vi "Read Roles.vi"(8 "error in (no error)":errorcluster, 11 "NormalGamePlayVSS in":refnum<class "NormalGamePlayVSS.lvclass">) -> (0 "error out":errorcluster, 2 "Roles":T1, 3 "NormalGamePlayVSS out":refnum<class "NormalGamePlayVSS.lvclass">)   [LabVIEW 2020, in "NormalGamePlayVSS.lvclass"]
uses:
  NormalGamePlayVSS.lvclass
  NormalAttackerRoleVSS_class/NormalAttackerRoleVSS.lvclass
  KeeperRoleVSS_class/KeeperRoleVSS.lvclass
  DefenderAreaRoleVSS_class/DefenderAreaRoleVSS.lvclass
  NormalGamePlayVSS.lvclass/NormalGamePlayVSS.ctl
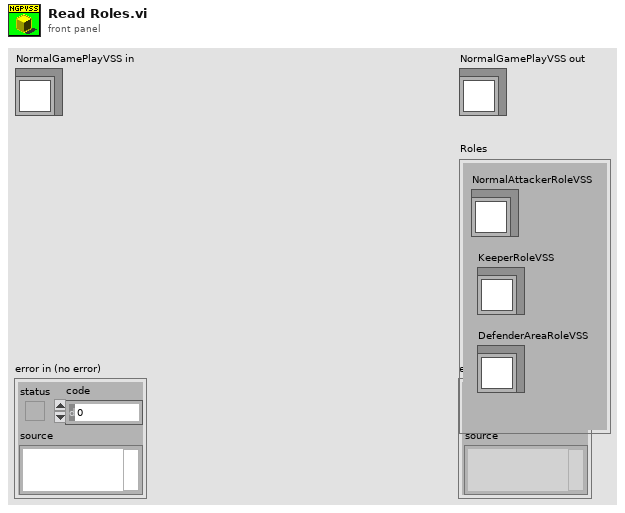
[diagram p1: front panel]
types:
  T1 = cluster{"NormalAttackerRoleVSS":refnum<class "NormalAttackerRoleVSS.lvclass">, "KeeperRoleVSS":refnum<class "KeeperRoleVSS.lvclass">, "DefenderAreaRoleVSS":refnum<class "DefenderAreaRoleVSS.lvclass">}
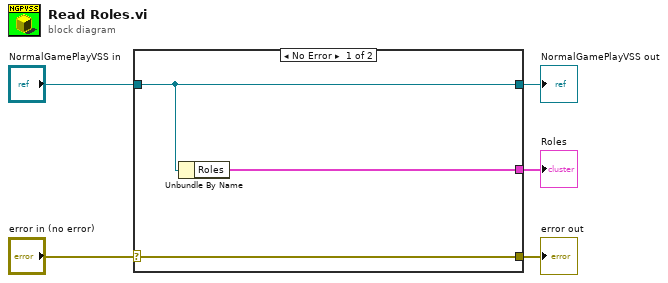
[diagram p0: block diagram]
diagram:
  n1 = case shown="No Error" "error in (no error)" {
    selector: "error in (no error)" -> [w8 w9]
    tunnel: [w8 w9] -> w4
    tunnel: [w7 w10] -> w2
    tunnel: "NormalGamePlayVSS in" -> [w7 w10]
    tunnel: [w6 _] -> w1
    frame No Error {
      n2 = Unbundle By Name(w7) -> ("Roles"=w6:T1)
    }
    frame Error {
    }
  }
  "error out" <- w4
  "NormalGamePlayVSS out" <- w2
  "Roles" <- w1
